vi "1D Fit Unscaled Weights.vi"(8 "error in (no error)":errorcluster, 9 "Weighted Fit":T1, 10 "Normalization Factor":dbl, 11 "Data Array":dbl[](array[numeric])) -> (0 "error out":errorcluster, 3 "Scaled Weight Array":dbl[](array[numeric]))   [LabVIEW 2021, in "Fits.lvlib"]
doc: "Computes Chi^2 weights for a normalized data array, by first unscaling the data and then rescaling the weights."
uses:
  Fits.lvlib
  IRF(X)PSED/Fit Weights Type v2.ctl
panel:
  # "see the AlliGator License on the block diagram (Ctrl+E or Window:Show Block Diagram)"
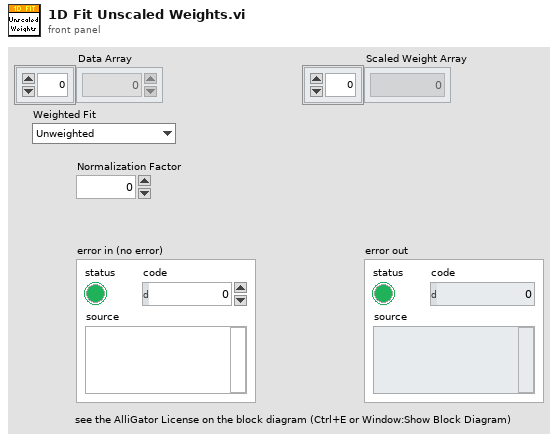
[diagram p1: front panel]
types:
  T1 = typedef "Fits.lvlib/Fit Weights Type v2.ctl" = enum16{"Unweighted", "1/Variance (Neyman)", "1/Variance (Pearson)", "Best of All"}
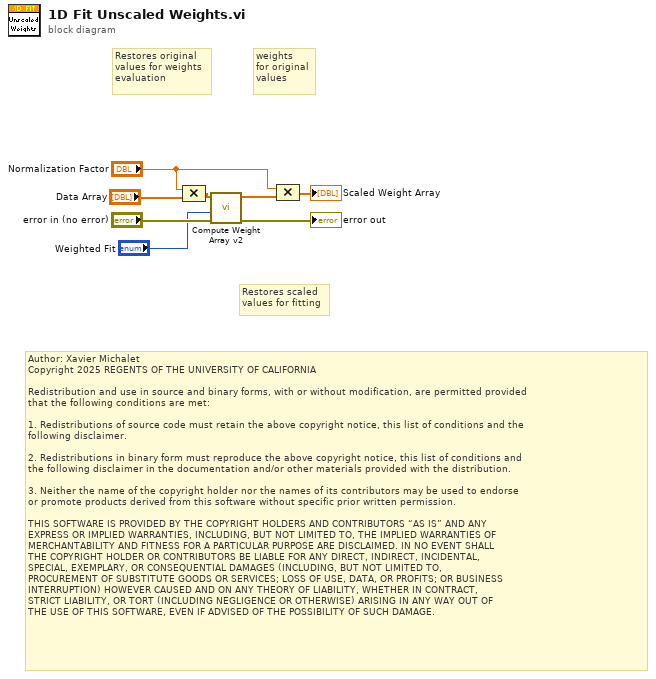
[diagram p0: block diagram]
diagram:
  # "weights\nfor original\nvalues"
  # "Author: Xavier Michalet\nCopyright 2025 REGENTS OF THE UNIVERSITY OF CALIFORNIA\n\nRedistribution and use in source and binary forms, with or without modification, are permitted provided\nthat the following conditions are met:\n\n1. Redistributions of source code must retain the above copyright notice, this list of conditions and the\nfollowing disclaimer.\n\n2. Redistributions in binary form must reproduce the above copyright notice, this list of conditions and\nthe following disclaimer in the documentation and/or other materials provided with the distribution.\n\n3. Neither the name of the copyright holder nor the names of its contributors may be used to endorse \nor promote products derived from this software without specific prior written permission.\n\nTHIS SOFTWARE IS PROVIDED BY THE COPYRIGHT HOLDERS AND CONTRIBUTORS “AS IS” AND ANY \nEXPRESS OR IMPLIED WARRANTIES, INCLUDING, BUT NOT LIMITED TO, THE IMPLIED WARRANTIES OF\nMERCHANTABILITY AND FITNESS FOR A PARTICULAR PURPOSE ARE DISCLAIMED. IN NO EVENT SHALL\nTHE COPYRIGHT HOLDER OR CONTRIBUTORS BE LIABLE FOR ANY DIRECT, INDIRECT, INCIDENTAL, \nSPECIAL, EXEMPLARY, OR CONSEQUENTIAL DAMAGES (INCLUDING, BUT NOT LIMITED TO, \nPROCUREMENT OF SUBSTITUTE GOODS OR SERVICES; LOSS OF USE, DATA, OR PROFITS; OR BUSINESS\nINTERRUPTION) HOWEVER CAUSED AND ON ANY THEORY OF LIABILITY, WHETHER IN CONTRACT, \nSTRICT LIABILITY, OR TORT (INCLUDING NEGLIGENCE OR OTHERWISE) ARISING IN ANY WAY OUT OF\nTHE USE OF THIS SOFTWARE, EVEN IF ADVISED OF THE POSSIBILITY OF SUCH DAMAGE."
  # "Restores scaled\nvalues for fitting"
  # "Restores original\nvalues for weights\nevaluation"
  n1 = Compound Arithmetic op=MULTIPLY("Normalization Factor", "Data Array") -> (w7:dbl[])
  n2 = call "Compute Weight Array v2.vi"("Error In"="error in (no error)", "Weighted Fit"="Weighted Fit", "Data Array"=w7) -> ("Error Out"=→"error out":errorcluster, "Weight Array"=w4:dbl[])  [unwired: 7 in]
  n3 = Compound Arithmetic op=MULTIPLY("Normalization Factor", w4) -> (→"Scaled Weight Array":dbl[])
